vi "teszt.vi"() -> ()   [LabVIEW 2023]
uses:
  <vilib>/regexp/Match Regular Expression.xnode
panel:
  out "submatch 3":string
  out "submatch 2":string
  out "submatch 1":string
  out "offset past match":i32
  out "after match":string
  out "whole match":string
  out "before match":string
  in  "multiline? (F)":bool
  in  "ignore case? (F)":bool
  in  "offset (0)":i32
  in  "string":string
  out "selection":bool
  out "PSRR (dB)":i32
  out "error out":errorcluster
  in  "error in":errorcluster
  in  "Boolean":bool
  # "^(Synchronous_PSRR_Meter\\.vi<ERR>|Synchronous_PSRR_Meter\\.vi<APPEND>)\\s*(.*?)\\s*(<b>Complete call chain:</b>.*)$"
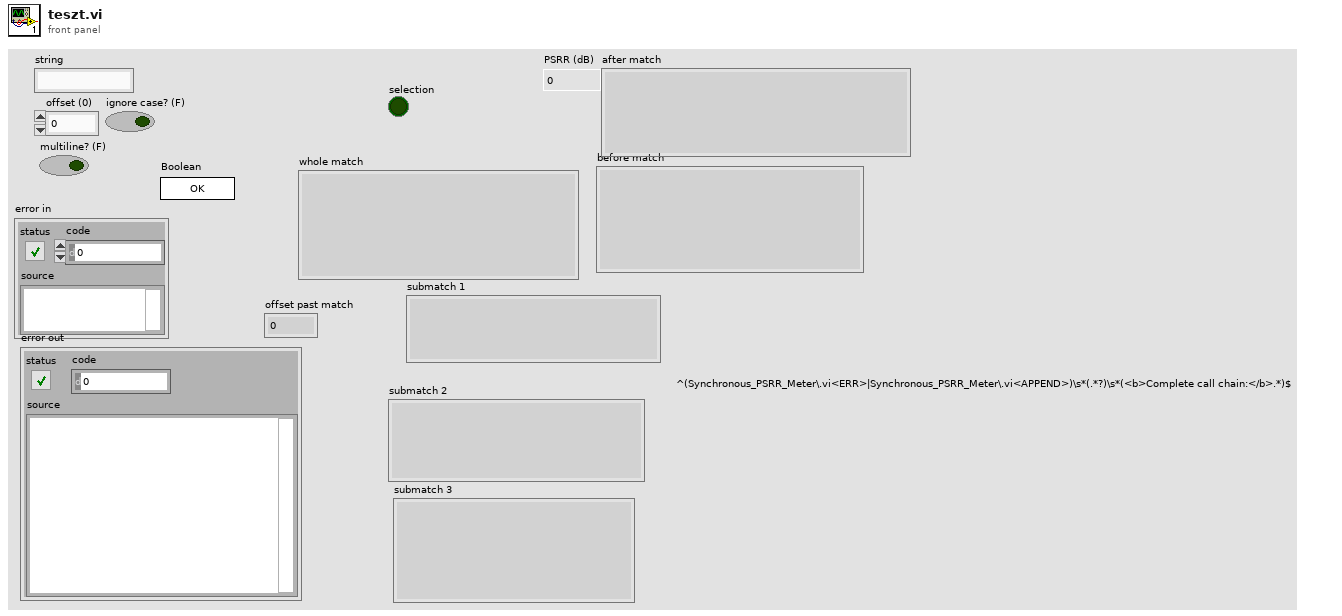
[diagram p1: front panel]
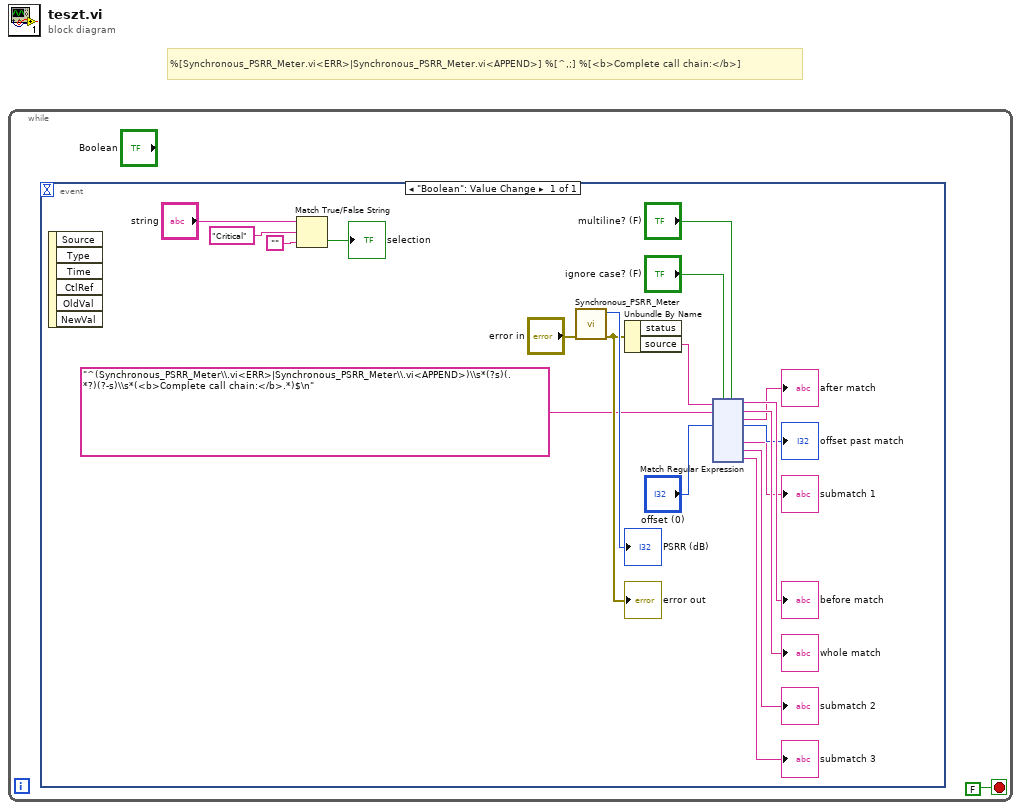
[diagram p0: block diagram]
diagram:
  # "%[Synchronous_PSRR_Meter.vi<ERR>|Synchronous_PSRR_Meter.vi<APPEND>] %[^,;] %[<b>Complete call chain:</b>]"
  n1 = while {
    stop <- FALSE stop-if-true
    n2 = event shown="[0] \"Boolean\": Value Change" {
      selector: _ -> [_]
      dyn-events: _ -> [_]
      timeout: _ -> [_]
      event "Boolean": Value Change {
        n3 = event-data() -> ()  [unwired: 1 in, 6 out]
        n4 = Match True/False String(2:"", 3:"Critical" ("true string"), 4:"string") -> (0:→"selection":bool)  [unwired: 1 out]
        n5 = call "Synchronous_PSRR_Meter.vi"("error in"="error in") -> ("error out"=w17:errorcluster, "PSRR (dB)"=→"PSRR (dB)":i32)  [unwired: 9 in]
        "error out" <- w17
        n6 = Unbundle By Name(w17) -> ("source"=w13:string)  [unwired: 1 out]
        n7 = xnode "Match Regular Expression"("input string"=w13, "regular expression"="^(Synchronous_PSRR_Meter\\.vi<ERR>|Synchronous_PSRR_Meter\\.vi<APPEND>)\\s*(?s)(.*?)(?-s)\\s*(<b>Complete call chain:</b>.*)$\n", "offset (0)"="offset (0)", "ignore case? (F)"="ignore case? (F)", "multiline? (F)"="multiline? (F)") -> ("before match"=→"before match":string, "whole match"=→"whole match":string, "after match"=→"after match":string, "offset past match"=→"offset past match":i32, "submatch 1"=→"submatch 1":string, "submatch 2"=→"submatch 2":string, "submatch 3"=→"submatch 3":string)  [unwired: 1 in, 1 out]
      }
    }
  }
